vi "Perform Measurements.vi"(7 "error in":errorcluster, 8 "Load Current":dbl, 9 "Nominal output voltage":dbl, 10 "State data":T2) -> (0 "error out":errorcluster, 1 "Measurement Results":T1, 2 "Load out":refnum<k15>, 3 "Source out":refnum<k15>)   [LabVIEW 2021, in "Scalar Efficiency And Load Regulation_PMIC.lvlib"]
uses:
  Scalar Efficiency And Load Regulation_PMIC.lvlib
  Measurement Results.ctl
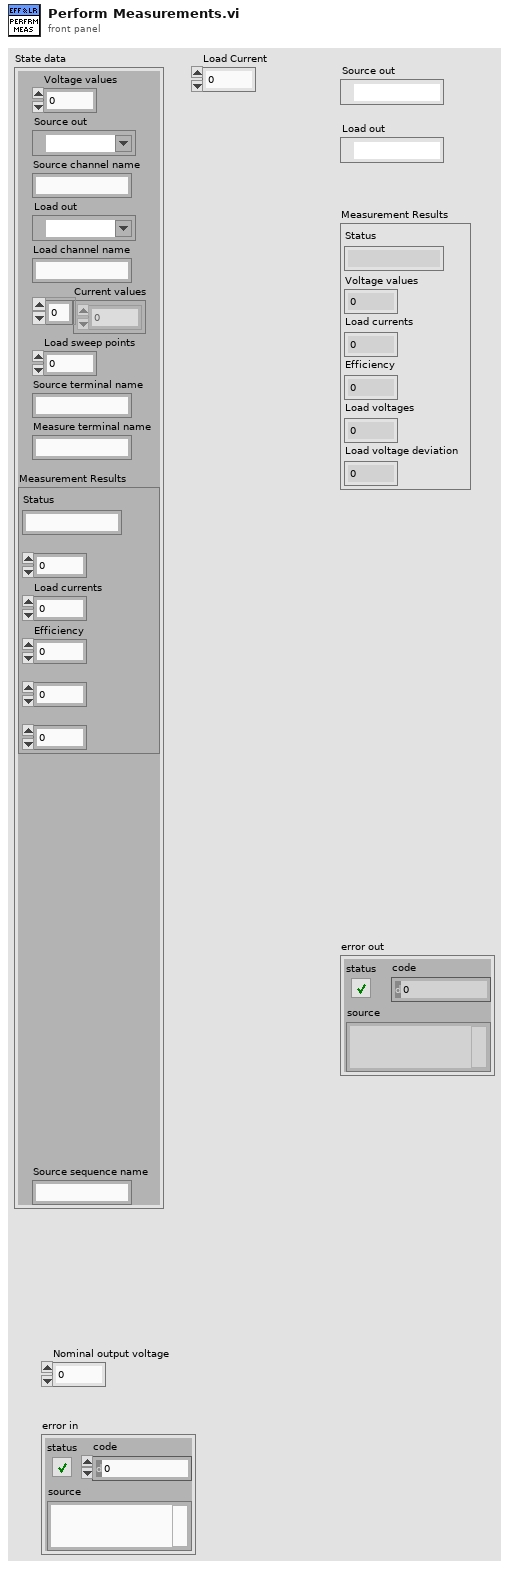
[diagram p1: front panel]
types:
  T1 = typedef "Scalar Efficiency And Load Regulation_PMIC.lvlib/Measurement Results.ctl" = cluster{"Status":string, "Voltage values":dbl, "Load currents":dbl, "Efficiency":dbl, "Load voltages":dbl, "Load voltage deviation":dbl}
  T2 = cluster{"Voltage values":dbl, "Source out":refnum<k15>, "Source channel name":string, "Load out":refnum<k15>, "Load channel name":string, "Current values":dbl[], "Load sweep points":i32, "Source terminal name":string, "Measure terminal name":string, "Measurement Results":T1, "Source sequence name":string}
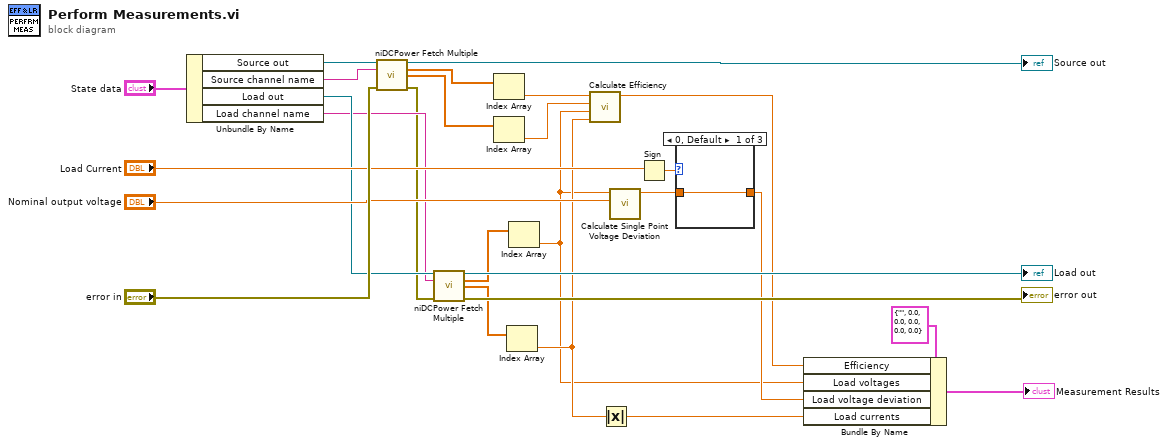
[diagram p0: block diagram]
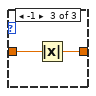
[diagram p3: hidden frame]
diagram:
  n1 = Unbundle By Name("State data") -> ("Source out"=w22:refnum<k15>, "Source channel name"=w21:string, "Load out"=w16:refnum<k15>, "Load channel name"=w15:string)
  n2 = call <instrlib>:"niDCPower Fetch Multiple.vi"("instrument handle"=w22, "channel name"=w21, "error in (no error)"="error in") -> ("instrument handle out"=→"Source out":refnum<k15>, "voltage measurements"=w13:dbl[], "current measurements"=w12:dbl[], "error out"=w14:errorcluster)  [unwired: 7 in, 2 out]
  n3 = call <instrlib>:"niDCPower Fetch Multiple.vi"("instrument handle"=w16, "channel name"=w15, "error in (no error)"=w14) -> ("instrument handle out"=→"Load out":refnum<k15>, "voltage measurements"=w9:dbl[], "current measurements"=w11:dbl[], "error out"=→"error out":errorcluster)  [unwired: 7 in, 2 out]
  n4 = Index Array(array=w13) -> (element=w2:dbl)  [unwired: 1 in]
  n5 = Index Array(array=w12) -> (element=w3:dbl)  [unwired: 1 in]
  n6 = Index Array(array=w11) -> (element=w4:dbl)  [unwired: 1 in]
  n7 = Index Array(array=w9) -> (element=w1:dbl)  [unwired: 1 in]
  n8 = call "Calculate Efficiency.vi"("load current measurements"=w4, "load voltage measurements"=w1, "source current measurements"=w3, "source voltage measurements"=w2) -> ("Efficiency(%)"=w10:dbl)  [unwired: 7 in]
  n9 = Absolute Value(x=w4) -> (abs(x)=w8:dbl)
  n10 = call "Calculate Single Point Voltage Deviation.vi"("Nominal output voltage"="Nominal output voltage", "Voltage measurements"=w1) -> ("Load voltage deviation"=w5:dbl)  [unwired: 9 in]
  n11 = Sign(1:"Load Current") -> (0:w6:dbl)
  n12 = case shown="0, Default" w6 {
    tunnel: [w28 w29 w31] -> w7
    tunnel: w5 -> [w28 w29 w30]
    frame 0, Default {
    }
    frame 1 {
    }
    frame -1 {
      n13 = Absolute Value(x=w30) -> (abs(x)=w31:dbl)
    }
  }
  n14 = Bundle By Name(cluster=T1 {"Status"="", "Voltage values"=0.0, "Load currents"=0.0, "Efficiency"=0.0, "Load voltages"=0.0, "Load voltage deviation"=0.0} ("Measurement Results"), "Efficiency"=w10, "Load voltages"=w1, "Load voltage deviation"=w7, "Load currents"=w8) -> (→"Measurement Results":T1)
